vi "global_channels.vi"() -> ()   [LabVIEW 2018]
panel:
  in  "Generator COM port":refnum<visa-resource-name>="COM3"
  in  "AOM manual on/off":tag="Dev1/port2/line0"
  in  "AWG":refnum<visa-resource-name>="dhcp-192-033-100-118"
  in  "Quicksyn":refnum<visa-resource-name>="COM4"
  in  "Reference Counter":tag="Dev2/ctr1"
  in  "Gate":tag="Dev1/ctr3"
  in  "Gate input":tag="/Dev1/PFI15"
  in  "Counter clock":tag="/Dev1/100MHzTimebase"
  in  "DAQ trigger input":tag="/Dev1/PFI0"
  in  "DAQ trigger output":tag="Dev1/port0/line1"
  in  "Counter trigger input":tag="/Dev1/PFI0"
  in  "Counter":tag="Dev1/ctr0"
  in  "Counter input":tag="/Dev1/PFI8"
  in  "Counter prescaler":u16(ring) items=["1x", "2x", "8x"]
  in  "Tritor":refnum<visa-resource-name>="COM3"
  in  "Reference gate":tag="/Dev2/PFI38" caption="Trigger Source"
  in  "Signal gate":tag="/Dev2/PFI34" caption="Trigger Source"
  in  "Laser Control":tag="Dev1/ao3"
  in  "Set x":tag="Dev1/ao0"
  in  "Set z":tag="Dev1/ao2"
  in  "Set y":tag="Dev1/ao1"
  # "ctr0"
  # "PFI8"
  # "PFI0"
  # "ctr3"
  # "port0/line1"
  # "PFI15"
  # "PFI0"
  # "port2/line0\n(PFI8 on board 2)"
  # "(PFI38 is used as conuter trigger input for AWG)"
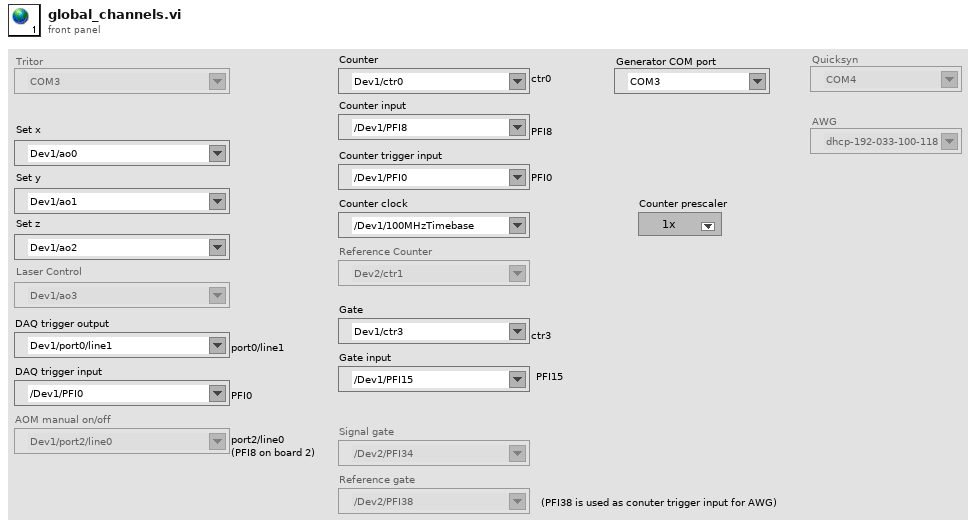
[diagram p1: front panel]
diagram:
